vi "ImpulseAnalyzer.vi"() -> ()   [LabVIEW 2015]
panel:
  out "XY Graph":cluster{dbl[], dbl[]}(graph)
  out "Array":dbl[][](array[numeric])
  in  "stop":bool
  in  "Time":dbl
  in  "Rate":dbl
  in  "Averages":dbl
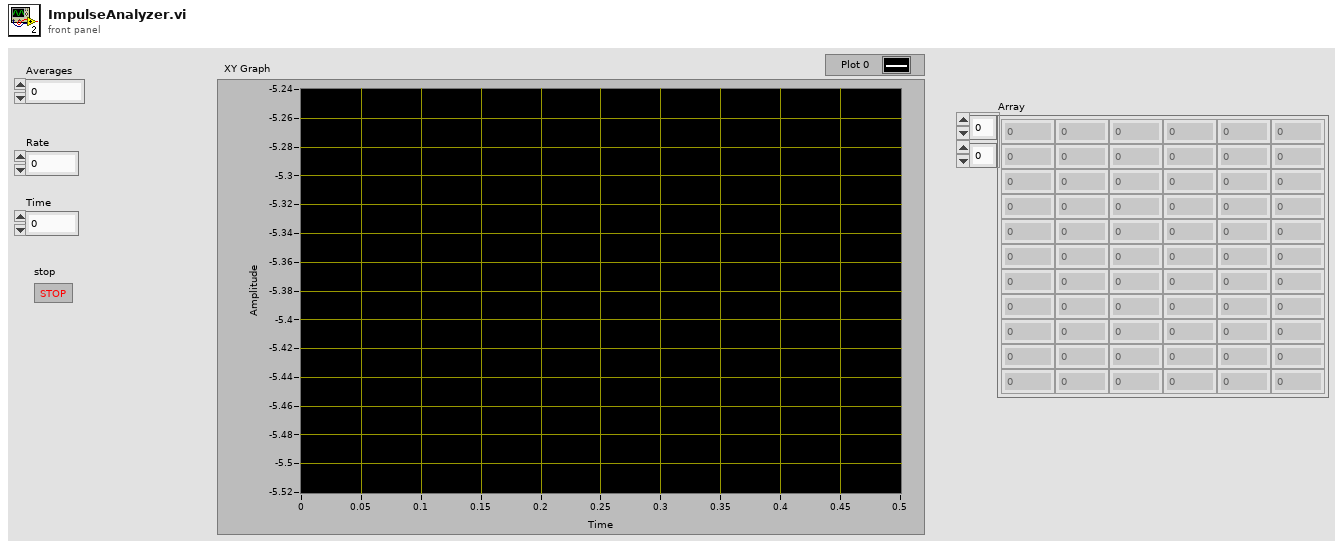
[diagram p1: front panel]
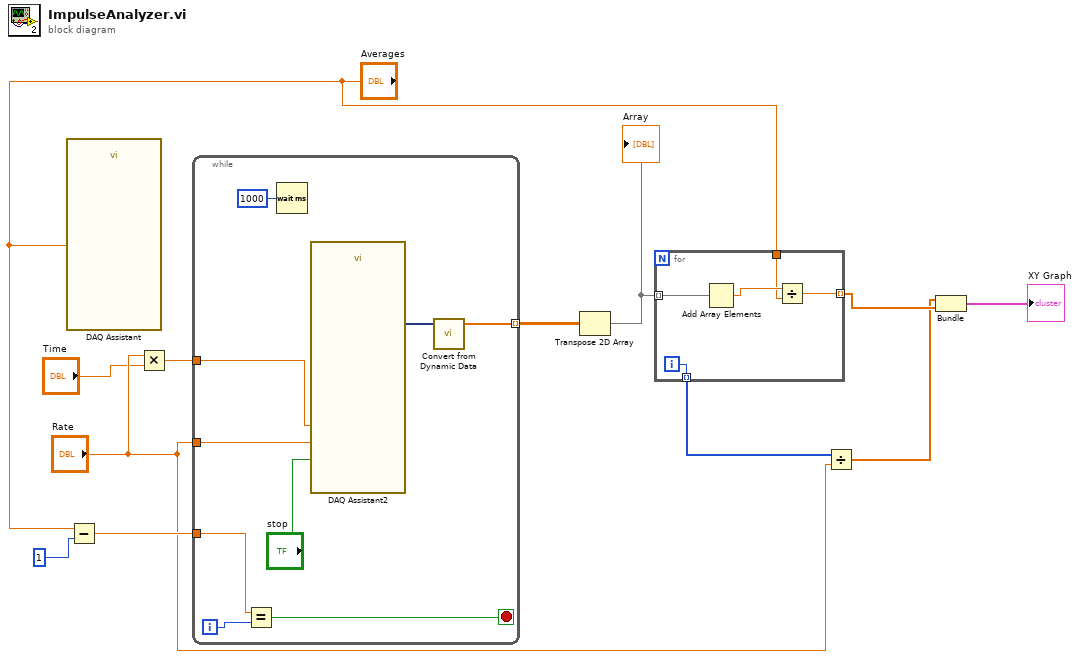
[diagram p0: block diagram]
diagram:
  n1 = call "DAQ Assistant"("number of samples"="Averages") -> ()  [unwired: 17 in, 2 out]
  n2 = Subtract(x="Averages", y=1) -> (x-y=w11:dbl)
  n3 = Multiply(x="Rate", y="Time") -> (x*y=w1:dbl)
  n4 = while {
    tunnel: w11 -> [w20]
    tunnel: [w16] -> w10 mode=indexing
    tunnel: "Rate" -> [w14]
    tunnel: w1 -> [w13]
    i -> [w19]
    stop <- w18 stop-if-true
    n5 = Equal?(x=w20, y=w19) -> (x = y?=w18:bool)
    n6 = Wait (ms)(milliseconds to wait=u32 1000) -> ()  [unwired: 1 out]
    n7 = call "DAQ Assistant2"("rate"=w14, "number of samples"=w13, "stop (F)"="stop") -> ("data"=w17:dynamicdata)  [unwired: 13 in, 3 out]
    n8 = call "Convert from Dynamic Data"("Dynamic Data Type"=w17) -> ("Array"=w16:dbl[])  [unwired: 3 in]
  }
  n9 = Transpose 2D Array(2D array=w10) -> (transposed array=w9:dbl[][])
  "Array" <- w9
  n10 = for {
    tunnel: w9 -> [w26] mode=indexing
    tunnel: "Averages" -> [w24]
    tunnel: [w23] -> w7 mode=indexing
    tunnel: [w22] -> w6 mode=indexing
    i -> [w22]
    n11 = Add Array Elements(numeric array=w26) -> (sum=w25:dbl)
    n12 = Divide(x=w25, y=w24) -> (x/y=w23:dbl)
  }
  n13 = Divide(x=w6, y="Rate") -> (x/y=w5:dbl[])
  n14 = Bundle(w5, w7) -> (→"XY Graph":cluster{dbl[], dbl[]})  [unwired: 1 in]
